vi "getLineFromTwoPoints.vi"(7 "x informed (optional)":dbl format="%#_13g", 8 "error in (no error)":errorcluster, 9 "Point 2":dbl[](array[numeric]), 10 "Point 1":dbl[](array[numeric]), 11 "Utilities in":refnum<class "Utilities.lvclass">) -> (0 "error out":errorcluster, 1 "linear coef":dbl, 2 "angular coef":dbl, 3 "Utilities out":refnum<class "Utilities.lvclass">, 5 "y to x informed (opitional)":dbl)   [LabVIEW 2020, in "Utilities.lvclass"]
uses:
  Utilities.lvclass
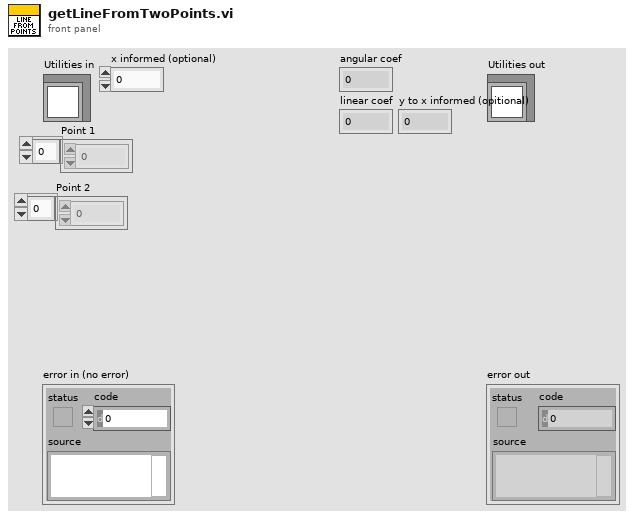
[diagram p1: front panel]
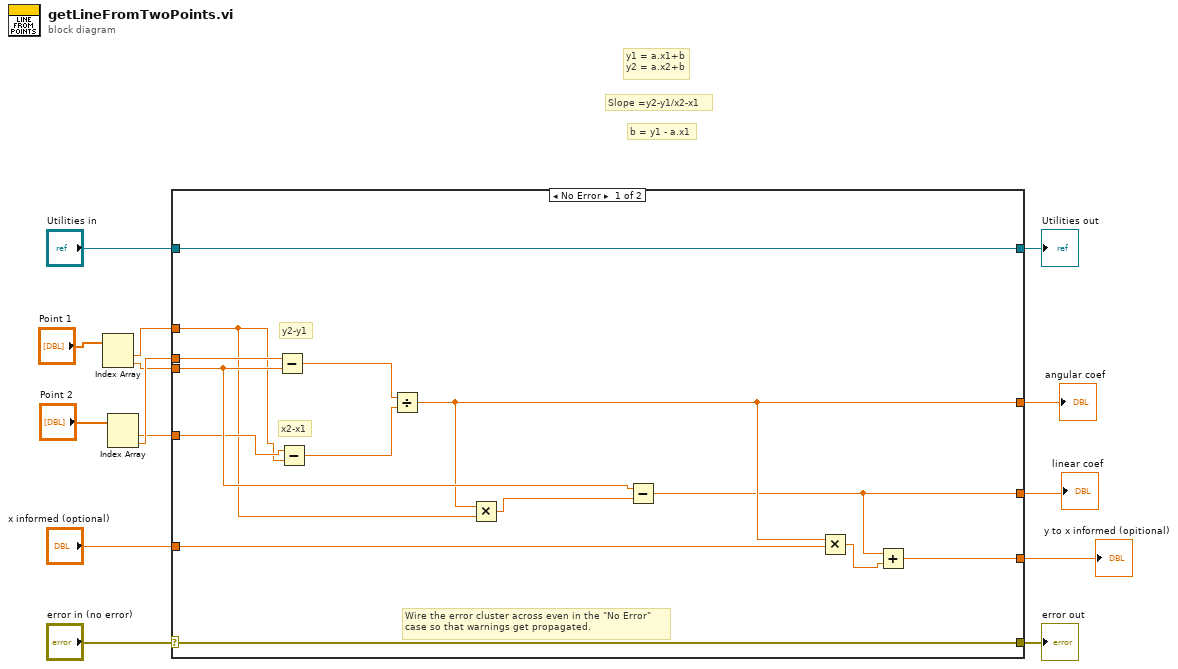
[diagram p0: block diagram]
diagram:
  # "b = y1 - a.x1"
  # "y1 = a.x1+b\ny2 = a.x2+b"
  # "Slope =y2-y1/x2-x1"
  n1 = Index Array(array="Point 1") -> (element #1=w5:dbl, element #2=w7:dbl)  [unwired: 2 in]
  n2 = Index Array(array="Point 2") -> (element #1=w6:dbl, element #2=w8:dbl)  [unwired: 2 in]
  n3 = case shown="No Error" "error in (no error)" {
    selector: "error in (no error)" -> [w27 w30]
    tunnel: [w27 w30] -> w13
    tunnel: [w28 w29] -> w11
    tunnel: "Utilities in" -> [w28 w29]
    tunnel: w8 -> [w26 _]
    tunnel: w7 -> [w23 _]
    tunnel: w6 -> [w21 _]
    tunnel: w5 -> [w20 _]
    tunnel: [w18 _] -> w4
    tunnel: [w16 _] -> w3
    tunnel: "x informed (optional)" -> [w19 _]
    tunnel: [w15 _] -> w1
    frame No Error {
      # "x2-x1"
      # "y2-y1"
      # "Wire the error cluster across even in the \"No Error\"\ncase so that warnings get propagated."
      n4 = Subtract(x=w26, y=w23) -> (x-y=w25:dbl)
      n5 = Subtract(x=w21, y=w20) -> (x-y=w24:dbl)
      n6 = Divide(x=w25, y=w24) -> (x/y=w18:dbl)
      n7 = Multiply(x=w18, y=w20) -> (x*y=w22:dbl)
      n8 = Subtract(x=w23, y=w22) -> (x-y=w16:dbl)
      n9 = Multiply(x=w18, y=w19) -> (x*y=w17:dbl)
      n10 = Add(x=w16, y=w17) -> (x+y=w15:dbl)
    }
    frame Error {
    }
  }
  "error out" <- w13
  "Utilities out" <- w11
  "angular coef" <- w4
  "linear coef" <- w3
  "y to x informed (opitional)" <- w1
